vi "_Replace Configuration Table By ID(Array).vi"(6 "Comment Express Pattern(^#)":string="^#", 8 "Error in":errorcluster caption="Error in (no error)", 9 "ID Col":i32, 10 "New Line":string[][](array[string]), 11 "Table in":string[][](array[string])) -> (0 "Error out":errorcluster, 3 "Table out":string[][](array[string]))   [LabVIEW 2017]
uses:
  e65b13f6-8d59-4e06-8efc-1876d752ea9f.vi
  e65b13f6-8d59-4e06-8efc-1876d752ea9f.vi/eb2405bd-5b2e-436b-9bb3-692ecf4a9268.vi
  e65b13f6-8d59-4e06-8efc-1876d752ea9f.vi/c8ad12e3-5e6d-40e1-92e0-1426ef45ec41.vi
  e65b13f6-8d59-4e06-8efc-1876d752ea9f.vi/effcbc1a-e97c-42d4-b61f-d821de102707.vi
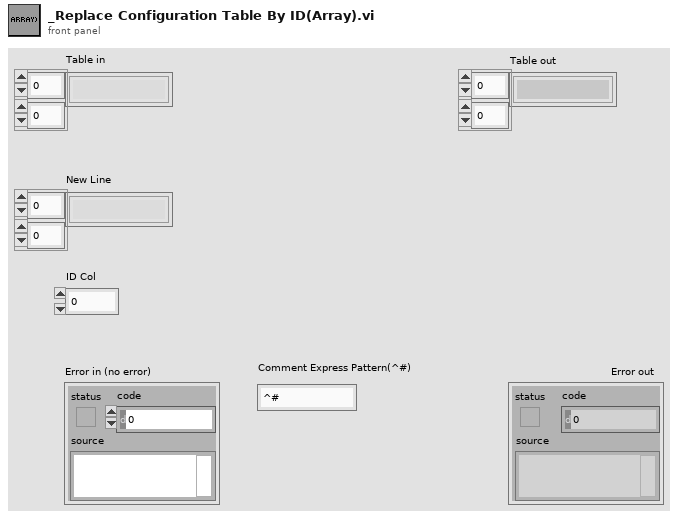
[diagram p1: front panel]
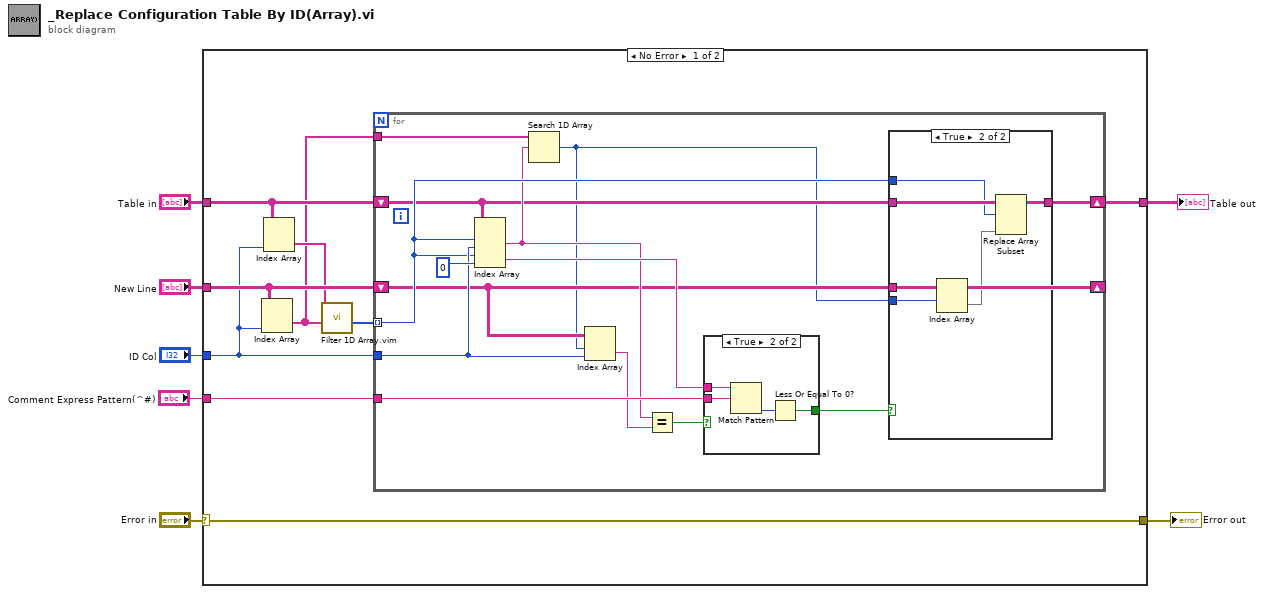
[diagram p0: block diagram]
diagram:
  n1 = case shown="No Error" "Error in" {
    selector: "Error in" -> [w14 w43]
    tunnel: "New Line" -> [w12 _]
    tunnel: "ID Col" -> [w9 _]
    tunnel: "Comment Express Pattern(^#)" -> [w16 _]
    tunnel: [w15 w42] -> w4
    tunnel: "Table in" -> [w13 w42]
    tunnel: [w14 w43] -> w1
    frame No Error {
      n2 = Index Array(array=w12, index (col)=w9) -> (element=w8:string[])  [unwired: 1 in]
      n3 = Index Array(array=w13, index (col)=w9) -> (element=w11:string[])  [unwired: 1 in]
      n4 = call "Filter 1D Array.vim"("items to filter"=w8, "array"=w11) -> ("filtered item indices"=w10:i32[])  [unwired: 4 in, 1 out]
      n5 = for {
        shift-right: [w27] -> w15
        shift-left: w13 -> [w18]
        tunnel: w16 -> [w29]
        shift-right: [w19] -> _
        shift-left: w12 -> [w19]
        tunnel: w10 -> [w26] mode=indexing
        tunnel: w9 -> [w28]
        tunnel: w8 -> [w21]
        n6 = Index Array(array=w18, index (row) #1=w26, index (col) #1=w28, index (row) #2=w26, index (col) #2=0) -> (element #1=w20:string, element #2=w23:string)
        n7 = Search 1D Array(1D array=w21, element=w20) -> (index of element=w17:i32)  [unwired: 1 in]
        n8 = Index Array(array=w19, index (row)=w17, index (col)=w28) -> (element=w24:string)
        n9 = Equal?(x=w20, y=w24) -> (x = y?=w22:bool)
        n10 = case shown="True" w22 {
          tunnel: w23 -> [_ w34]
          tunnel: w29 -> [_ w33]
          tunnel: [_ w31] -> w25
          frame False {
          }
          frame True {
            n11 = Match Pattern(string=w34, regular expression=w33) -> (offset past match=w32:i32)  [unwired: 1 in, 3 out]
            n12 = Less Or Equal To 0?(x=w32) -> (x <= 0?=w31:bool)
          }
        }
        n13 = case shown="True" w25 {
          tunnel: w18 -> [w35 w41]
          tunnel: [w35 w40] -> w27
          tunnel: w19 -> [_ w39]
          tunnel: w26 -> [_ w38]
          tunnel: w17 -> [_ w36]
          frame False {
          }
          frame True {
            n14 = Index Array(array=w39, index (row)=w36) -> (element=w37:string[])  [unwired: 1 in]
            n15 = Replace Array Subset(array=w41, new element=w37, index (row)=w38) -> (w40:string[][])  [unwired: 1 in]
          }
        }
      }
    }
    frame Error {
    }
  }
  "Table out" <- w4
  "Error out" <- w1
